vi "Flyhwheel_Lookup.vi"() -> (1 "Flywheel_Lookup_Table":dbl[][](array[numeric]))   [LabVIEW 2019]
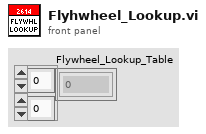
[diagram p1: front panel]
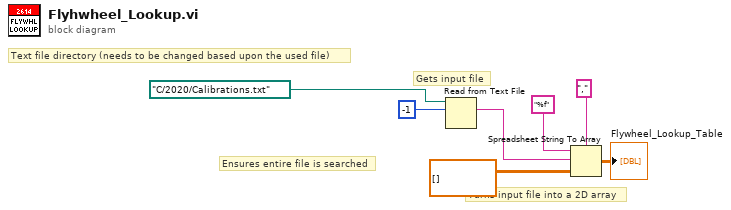
[diagram p0: block diagram]
diagram:
  # "Ensures entire file is searched"
  # "Gets input file"
  # "Turns input file into a 2D array"
  # "Text file directory (needs to be changed based upon the used file)"
  n1 = Read from Text File(file (use dialog)=path "C:/2020/Calibrations.txt", count=-1) -> (text=w3:string)  [unwired: 2 in, 3 out]
  n2 = Spreadsheet String To Array(delimiter (Tab)=",", format string="%f", spreadsheet string=w3, array type (2D Dbl)=dbl[][] []) -> (array=→"Flywheel_Lookup_Table":dbl[][])
